vi "Change status of valves3 boxes 32bit.vi"(6 "error in Box ID1":errorcluster, 7 "error in Box ID2":errorcluster, 8 "error in Box ID0":errorcluster, 9 "Status of inlets and\non-chip valves":bool[](array[boolean]), 10 "Box # & Valve #":cluster{i32[], i32[]}, 11 "Box # => Box ID":i32[](array[numeric])) -> (0 "error out Box ID1":errorcluster, 1 "error out Box ID0":errorcluster, 2 "Valve box ID1":bool[](array[boolean]), 3 "Valve box ID0":bool[](array[boolean]), 4 "error out Box ID2":errorcluster, 5 "Valve box ID2":bool[](array[boolean]))   [LabVIEW 2014]
uses:
  Automation/PacDrive/PacDrive.dll
panel:
  # "Box #1 -> ID"
  # "Box #2 -> ID"
  # "Box #3 -> ID"
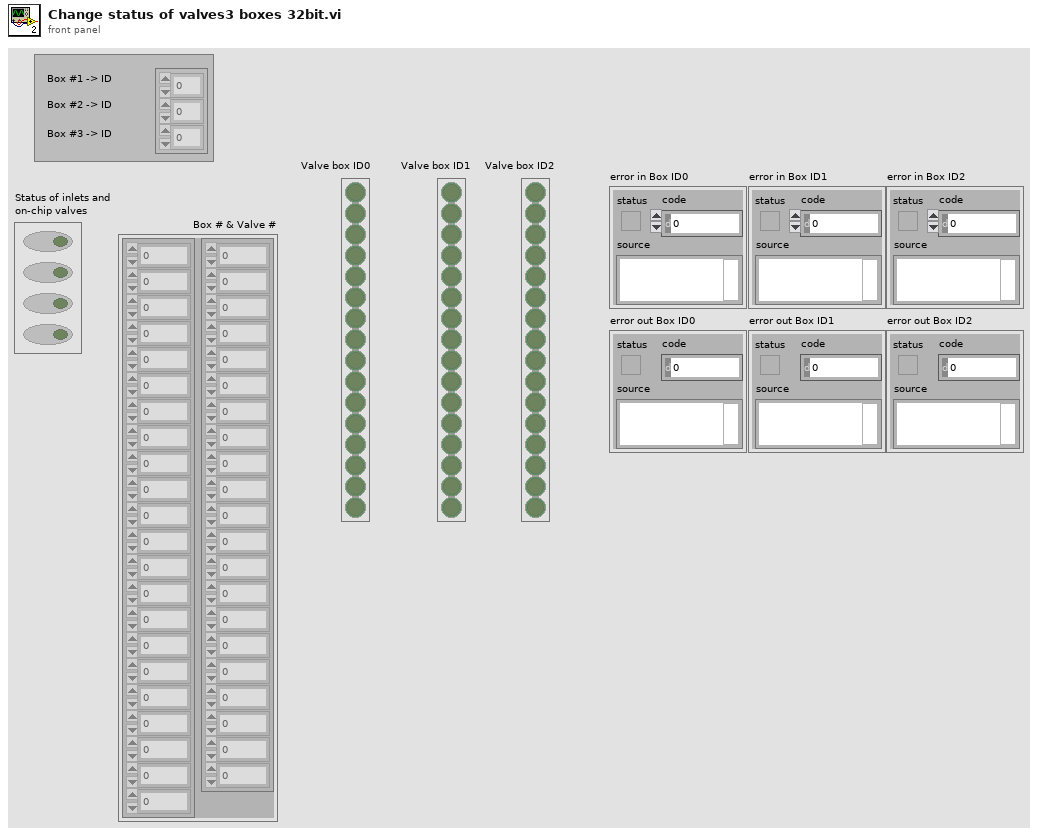
[diagram p1: front panel]
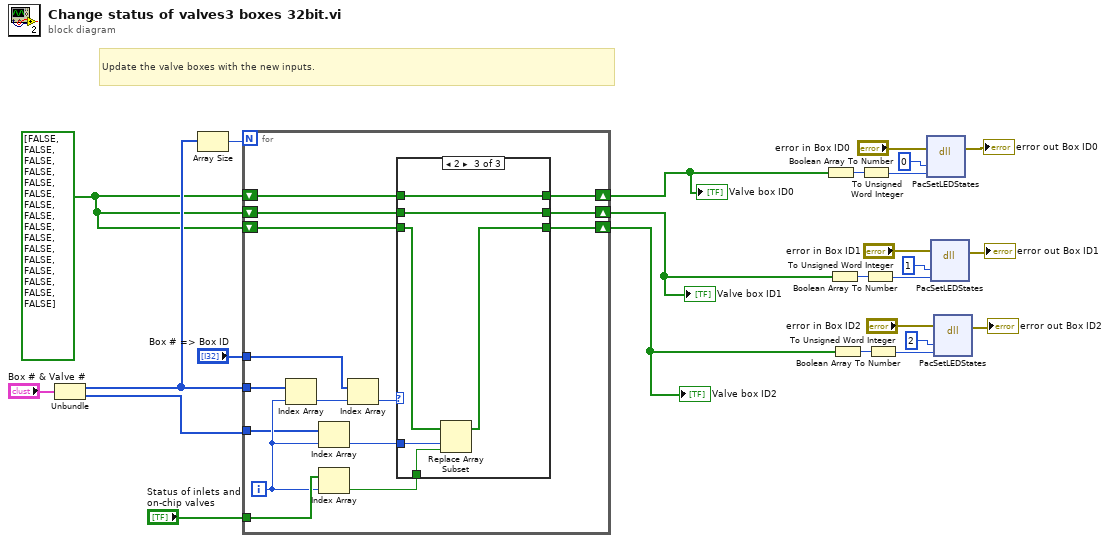
[diagram p0: block diagram]
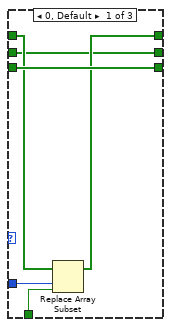
[diagram p2: hidden frame]
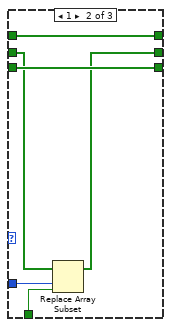
[diagram p3: hidden frame]
diagram:
  w9 = bool[] [FALSE, FALSE, FALSE, FALSE, FALSE, FALSE, FALSE, FALSE, FALSE, FALSE, FALSE, FALSE, FALSE, FALSE, FALSE, FALSE]
  # "Update the valve boxes with the new inputs."
  n1 = Unbundle("Box # & Valve #") -> (w23:i32[], w24:i32[])
  n2 = Array Size(array=w23) -> (size(s)=w22:i32)
  n3 = for {
    N: w22 -> [_]
    tunnel: "Status of inlets and\non-chip valves" -> [w40]
    shift-right: [w28] -> w1
    shift-left: w9 -> [w35]
    shift-right: [w27] -> w2
    shift-left: w9 -> [w34]
    tunnel: w23 -> [w37]
    tunnel: w24 -> [w36]
    tunnel: "Box # => Box ID" -> [w31]
    shift-right: [w26] -> w3
    shift-left: w9 -> [w30]
    i -> [w38]
    n4 = Index Array(array=w37, index=w38) -> (element=w32:i32)
    n5 = Index Array(array=w36, index=w38) -> (element=w33:i32)
    n6 = Index Array(array=w40, index=w38) -> (element=w39:bool)
    n7 = Index Array(array=w31, index=w32) -> (element=w29:i32)
    n8 = case shown="2" w29 {
      tunnel: w39 -> [w46 w52 w58]
      tunnel: w33 -> [w45 w51 w57]
      tunnel: w35 -> [w43 w50 w55]
      tunnel: [w42 w50 w55] -> w28
      tunnel: w34 -> [w41 w48 w56]
      tunnel: [w41 w47 w56] -> w27
      tunnel: w30 -> [w44 w49 w54]
      tunnel: [w44 w49 w53] -> w26
      frame 0, Default {
        n9 = Replace Array Subset(array=w43, new element=w46, index=w45) -> (w42:bool[])
      }
      frame 1 {
        n10 = Replace Array Subset(array=w48, new element=w52, index=w51) -> (w47:bool[])
      }
      frame 2 {
        n11 = Replace Array Subset(array=w54, new element=w58, index=w57) -> (w53:bool[])
      }
    }
  }
  "Valve box ID2" <- w3
  "Valve box ID1" <- w2
  "Valve box ID0" <- w1
  n12 = Boolean Array To Number(Boolean array=w1) -> (number=w19:u32)
  n13 = Boolean Array To Number(Boolean array=w2) -> (number=w18:u32)
  n14 = Boolean Array To Number(Boolean array=w3) -> (number=w4:u32)
  n15 = To Unsigned Word Integer(number=w19) -> (unsigned 16bit integer=w21:u16)
  n16 = To Unsigned Word Integer(number=w18) -> (unsigned 16bit integer=w16:u16)
  n17 = To Unsigned Word Integer(number=w4) -> (unsigned 16bit integer=w6:u16)
  n18 = dll-call lib="I:/Transfer/Marija/Automation/PacDrive/PacDrive.dll" fn="PacSetLEDStates"(error in="error in Box ID0", "PacNum"=0, "LEDStates"=w21) -> (error out=→"error out Box ID0":errorcluster)  [unwired: 5 in, 1 out]
  n19 = dll-call lib="I:/Transfer/Marija/Automation/PacDrive/PacDrive.dll" fn="PacSetLEDStates"(error in="error in Box ID1", "PacNum"=1, "LEDStates"=w16) -> (error out=→"error out Box ID1":errorcluster)  [unwired: 5 in, 1 out]
  n20 = dll-call lib="I:/Transfer/Marija/Automation/PacDrive/PacDrive.dll" fn="PacSetLEDStates"(error in="error in Box ID2", "PacNum"=2, "LEDStates"=w6) -> (error out=→"error out Box ID2":errorcluster)  [unwired: 5 in, 1 out]
